vi "manualAmp.vi"(10 "Use DDS display equivalent?":bool, 11 "Manual Amplitude (0-1)":dbl) -> (2 "DDS display value":u8, 3 "Amplitude string out":string)   [LabVIEW 2012, in "DDS9954_v2013.lvlib"]
uses:
  DDS9954_v2013.lvlib
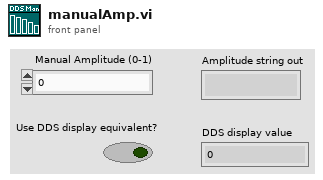
[diagram p1: front panel]
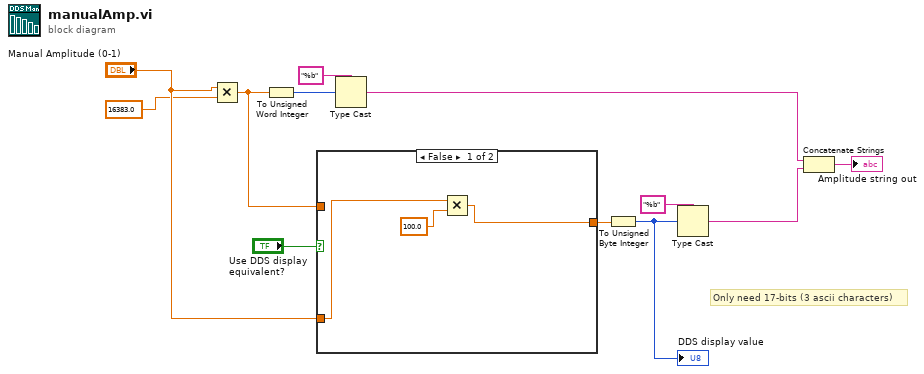
[diagram p0: block diagram]
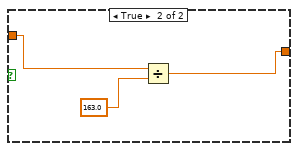
[diagram p2: hidden frame]
diagram:
  # "Only need 17-bits (3 ascii characters)"
  n1 = Multiply(x="Manual Amplitude (0-1)", y=16383.0) -> (x*y=w9:dbl)
  n2 = To Unsigned Word Integer(number=w9) -> (unsigned 16bit integer=w12:u16)
  n3 = case shown="False" "Use DDS display equivalent?" {
    tunnel: w9 -> [_ w18]
    tunnel: "Manual Amplitude (0-1)" -> [w15 _]
    tunnel: [w13 w16] -> w6
    frame False {
      n4 = Multiply(x=w15, y=100.0) -> (x*y=w13:dbl)
    }
    frame True {
      n5 = Divide(x=w18, y=163.0) -> (x/y=w16:dbl)
    }
  }
  n6 = Type Cast(type="%b", x=w12) -> (*(type *) &x=w5:string)
  n7 = To Unsigned Byte Integer(number=w6) -> (unsigned 8bit integer=w8:u8)
  "DDS display value" <- w8
  n8 = Type Cast(type="%b", x=w8) -> (*(type *) &x=w1:string)
  n9 = Concatenate Strings(w5, w1) -> (→"Amplitude string out":string)
